vi "Write Pulse Configuration.vi"(8 "error in (no error)":errorcluster, 10 "Configuration":T1={"Post-trigger delay"=0.01, "Post-trigger duration"=0.1, "Rate"=1000000.0, "Ranges"=[10.0], "Re-name channels"=[], "Active channels"="0:1", "External clock"=FALSE} {"Rate" format="%#_8pHz"; "Post-trigger duration" format="%#_6ps"; "Post-trigger delay" format="%#_6ps"; "Ranges" format="%#_6pV"}, 11 "DAQmx Synthesizer in":refnum<class "DAQmx Synthesizer.lvclass">) -> (0 "error out":errorcluster, 3 "DAQmx Synthesizer out":refnum<class "DAQmx Synthesizer.lvclass">)   [LabVIEW 2021, in "DAQmx Synthesizer.lvclass"]
uses:
  DAQmx Synthesizer.lvclass
  Instruments/Pulse Driver/Pusle Driver Configuration.ctl
  DAQmx Synthesizer.lvclass/DAQmx Synthesizer.ctl
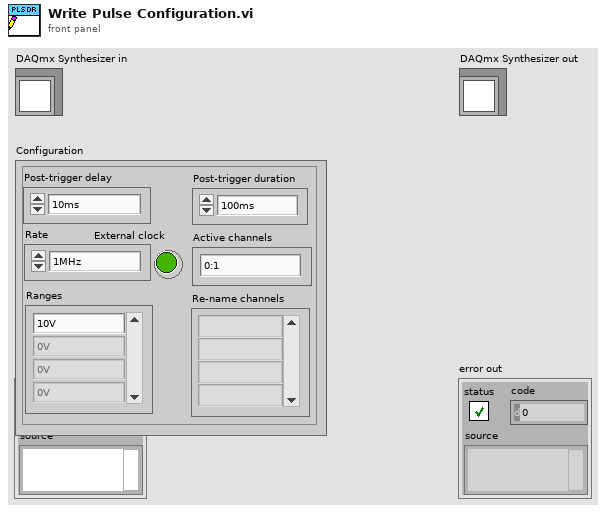
[diagram p1: front panel]
types:
  T1 = typedef "Pusle Driver Configuration.ctl" = cluster{"Post-trigger delay":dbl, "Post-trigger duration":dbl, "Rate":dbl, "Ranges":dbl[], "Re-name channels":string[], "Active channels":string, "External clock":bool}
  T2 = typedef "DAQmx Synthesizer Configuration.ctl" = cluster{"Channel names":string[], "Output channels":string, "Waveform file":path, "Offset":dbl, "Scale":dbl, "Ranges":dbl[], "Post-trigger delay":dbl, "Post-trigger duration":dbl, "Rate":dbl, "Re-name channels":string[], "Active channels":string, "External\nclock":bool}
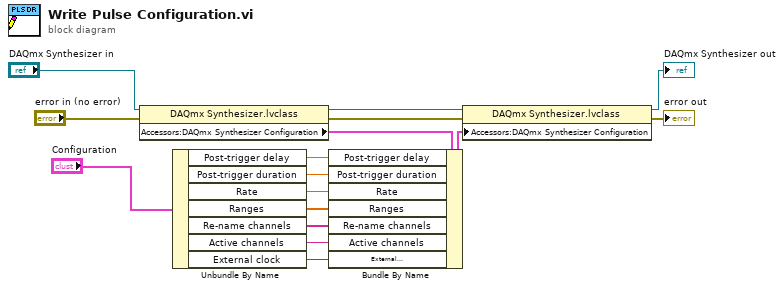
[diagram p0: block diagram]
diagram:
  n1 = property class="DAQmx Synthesizer.lvclass"(reference="DAQmx Synthesizer in", error in="error in (no error)") -> (reference out=w9:refnum<class "DAQmx Synthesizer.lvclass">, error out=w6:errorcluster, "Accessors:DAQmx Synthesizer Configuration"=w14:T2)
  n2 = Unbundle By Name("Configuration") -> ("Post-trigger delay"=w12:dbl, "Post-trigger duration"=w11:dbl, "Rate"=w5:dbl, "Ranges"=w4:dbl[], "Re-name channels"=w3:string[], "Active channels"=w2:string, "External clock"=w1:bool)
  n3 = Bundle By Name(cluster=w14, "Post-trigger delay"=w12, "Post-trigger duration"=w11, "Rate"=w5, "Ranges"=w4, "Re-name channels"=w3, "Active channels"=w2, "External\nclock"=w1) -> (w10:T2)
  n4 = property class="DAQmx Synthesizer.lvclass"(reference=w9, error in=w6, "Accessors:DAQmx Synthesizer Configuration"=w10) -> (reference out=→"DAQmx Synthesizer out":refnum<class "DAQmx Synthesizer.lvclass">, error out=→"error out":errorcluster)
